vi "string function.vi"() -> ()   [LabVIEW 2019]
panel:
  out "String 4":string
  in  "String 3":string="Day"
  in  "String 2":string="Mothers"
  in  "String  1":string="Happy"
  out "length":i32
  in  "String":string="Happy mothers day"
  # "STRING FUNCTION"
  # "1)String length"
  # "2) Concatenate string"
  # "\\.code display"
  # "Happy\\sMothers\\sDay\\s!!!\\s"
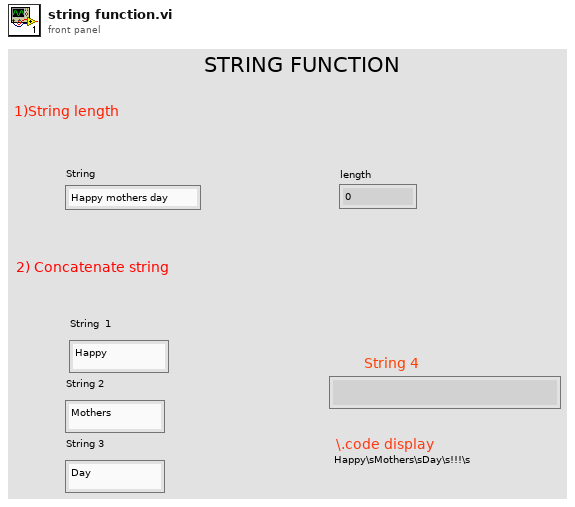
[diagram p1: front panel]
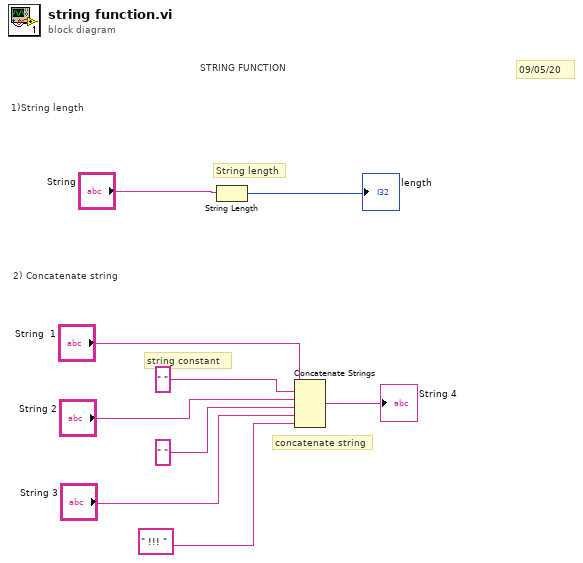
[diagram p0: block diagram]
diagram:
  # "09/05/20"
  # "string constant"
  # "concatenate string"
  # "2) Concatenate string"
  # "String length"
  # "STRING FUNCTION"
  # "1)String length"
  n1 = String Length(string="String") -> (length=→"length":i32)
  n2 = Concatenate Strings("String  1", " " ("concatenated string"), "String 2", " " ("concatenated string"), "String 3", " !!! " ("concatenated string")) -> (→"String 4":string)
